vi "Add Braces.vi"   [LabVIEW 2019, in "SMO.Transport.lvclass"]
uses:
  SMO.Transport.lvclass
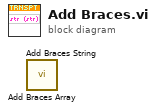
[diagram p0: block diagram]
diagram:
  n1 = call "Add Braces Array.vi"() -> ()  [unwired: 1 in, 1 out]
  n2 = call "Add Braces String.vi"() -> ()  [unwired: 1 in, 1 out]
